vi "Enk wykryj zmiany sygn.vi"(11 "Array in":dbl[](array[numeric])) -> (2 "l.probek":i32[](array[numeric]), 3 "skoki":dbl[](array[numeric]))   [LabVIEW 2014]
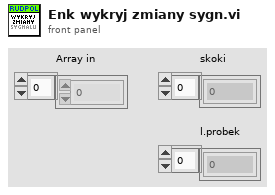
[diagram p1: front panel]
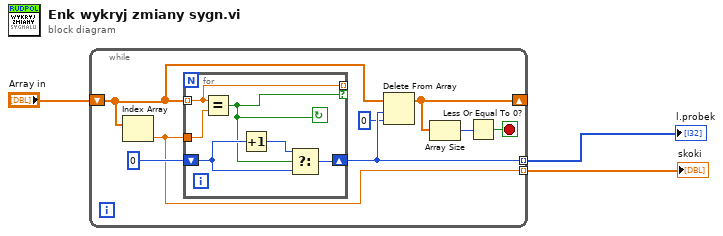
[diagram p0: block diagram]
diagram:
  n1 = while {
    shift-right: [w9] -> _
    shift-left: "Array in" -> [w10]
    tunnel: [w5] -> w2 mode=indexing
    tunnel: [w6] -> w1 mode=indexing
    stop <- w8 stop-if-true
    n2 = Index Array(array=w10) -> (element=w6:dbl)  [unwired: 1 in]
    n3 = for {
      tunnel: w10 -> [w13] mode=indexing
      tunnel: w6 -> [w17]
      shift-right: [w16] -> w5
      shift-left: 0 -> [w15]
      tunnel: [w13] -> _ mode=indexing if=w12
      stop <- w12 continue-if-true
      n4 = Equal?(x=w13, y=w17) -> (x = y?=w12:bool)
      n5 = Increment(x=w15) -> (x+1=w14:i32)
      n6 = Select(t=w14, s=w12, f=w15) -> (s? t:f=w16:i32)
    }
    n7 = Delete From Array(array=w10, length=w5, index=0) -> (array with subset deleted=w9:dbl[])  [unwired: 1 out]
    n8 = Array Size(array=w9) -> (size(s)=w7:i32)
    n9 = Less Or Equal To 0?(x=w7) -> (x <= 0?=w8:bool)
  }
  "l.probek" <- w2
  "skoki" <- w1
